vi "Start_ControlPowerRelay.vi"(8 "error in":errorcluster, 11 "ON - LC\nOFF - RS":bool) -> (0 "error out":errorcluster, 3 "ControlPowerRelayTaskOut":refnum<k21>)   [LabVIEW 2022 SP3]
doc: "This VI will start the control power relay task and command the relay. True - LC (Control Board Tests) ; False - RS-12 (Carrier Board Tests)"
uses:
  <vilib>/DAQmx/write.llb/DAQmx Write (Digital Bool 1Line 1Point).vi
  <vilib>/DAQmx/miscellaneous.llb/DAQmx Fill In Error Info.vi
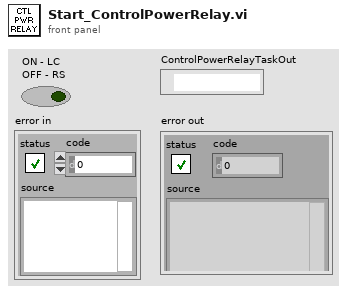
[diagram p1: front panel]
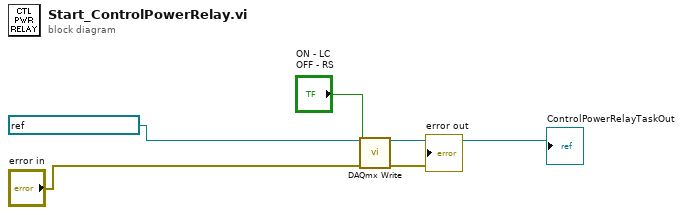
[diagram p0: block diagram]
diagram:
  n1 = call-poly <vilib>:"DAQmx Write.vi"("task/channels in"=refnum<k21> "BTS_ControlPower_Relay", "data"="ON - LC\nOFF - RS", "error in"="error in") -> ("task out"=→"ControlPowerRelayTaskOut":refnum<k21>, "error out"=→"error out":errorcluster)  [unwired: 10 in, 1 out]
